vi "Stop.vi"(8 "error in (no error)":errorcluster, 10 "Message in":refnum<class "StopMessage.lvclass">, 11 "StageSPIM in":refnum<class "StageSPIM.lvclass">) -> (0 "error out":errorcluster, 3 "StageSPIM out":refnum<class "StageSPIM.lvclass">)   [LabVIEW 2012, in "StageSPIM.lvclass"]
doc: "This member function is called when the statemachine in the run.vi receives an 'stop' command. It relays the message to all observers of the component.\n\nOverride this member function in your derived class if you need additional stop functionality (but don't forget to call the parent method)."
uses:
  StageSPIM.lvclass
  <vilib>/Distrio/Murmex/StopMessage/StopMessage.lvclass
  <vilib>/Distrio/Murmex/Murmex/Murmex.lvclass
  <vilib>/Distrio/Murmex/GenericMessage/GenericMessage.lvclass
  <vilib>/Distrio/Murmex/Message/Add or replace parameter.vi
panel:
  # "This method is called when the STOP\ntrigger is sent. \n\nOverride this method when your component needs to\nrespond to this trigger. \n\nCall parent for proper implementation"
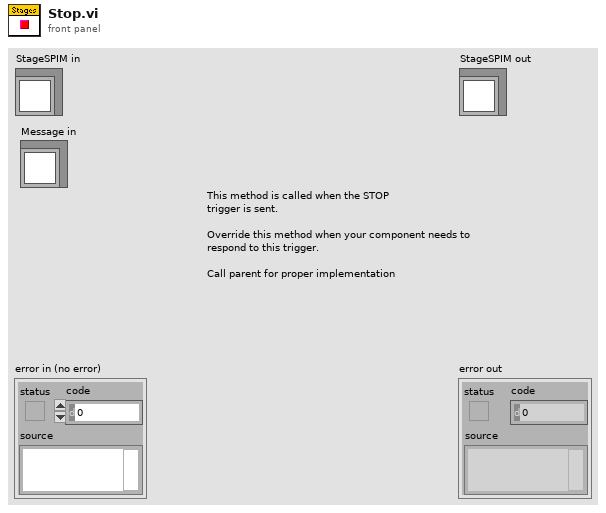
[diagram p1: front panel]
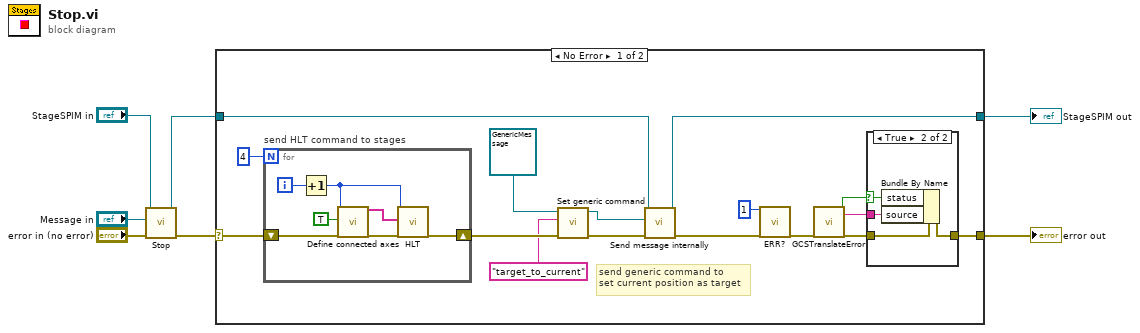
[diagram p0: block diagram]
diagram:
  n1 = call-parent "Stop.vi"("error in (no error)"="error in (no error)", "Message in"="Message in", "Murmex in"="StageSPIM in") -> ("error out"=w4:errorcluster, "Murmex out"=w3:refnum<class "StageSPIM.lvclass">)  [unwired: 7 in]
  n2 = case shown="No Error" w4 {
    selector: w4 -> [w23 w36]
    tunnel: w3 -> [w10 w37]
    tunnel: [w9 w37] -> w2
    tunnel: [w13 w36] -> w1
    frame No Error {
      # "send generic command to\nset current position as target"
      n3 = for "send HLT command to stages" {
        N: 4 -> [_]
        shift-right: [w35] -> w21
        shift-left: w23 -> [w32]
        i -> [w34]
        n4 = Increment(x=w34) -> (x+1=w31:i32)
        n5 = call "Define connected axes.vi"("System no."=w31, "Read from\ncontroller?"=TRUE ("Read from\ncontroller?"), "error in"=w32) -> ("Conn. Axes out"=w29:string[], "error out"=w33:errorcluster)  [unwired: 15 in]
        n6 = call "HLT.vi"("System no."=w31, "Affected axes"=w29, "error in"=w33) -> ("error out"=w35:errorcluster)  [unwired: 16 in]
      }
      n7 = call <vilib>:"Set generic command.vi"("error in (no error)"=w21, "generic command"="target_to_current", "GenericMessage in"=refnum<class "GenericMessage.lvclass"> refnum ("Distrio Murmex 1.2:GenericMessage")) -> ("error out"=w12:errorcluster, "GenericMessage out"=w8:refnum<class "GenericMessage.lvclass">)  [unwired: 7 in]
      n8 = call <vilib>:"Send message internally.vi"("error in (no error)"=w12, "Message"=w8, "Murmex in"=w10) -> ("error out"=w11:errorcluster, "Murmex out"=w9:refnum<class "StageSPIM.lvclass">)  [unwired: 7 in]
      n9 = call "ERR?.vi"("System no."=1, "error in"=w11) -> ("error out"=w14:errorcluster)  [unwired: 16 in, 1 out]
      n10 = call "GCSTranslateError.vi"("error in"=w14) -> ("GCS Error?"=w17:bool, "Error Description"=w18:string, "error out"=w16:errorcluster)  [unwired: 16 in]
      n11 = case shown="True" w17 {
        selector: w17 -> [_ w26]
        tunnel: w16 -> [w24 w28]
        tunnel: [w24 w27] -> w13
        tunnel: w18 -> [_ w25]
        frame False {
        }
        frame True {
          n12 = Bundle By Name(cluster=w28, "status"=w26, "source"=w25) -> (w27:errorcluster)
        }
      }
    }
    frame Error {
    }
  }
  "error out" <- w1
  "StageSPIM out" <- w2
